vi "Configure Lister.vi"(8 "error in (no error)":errorcluster, 10 "Serial Bus Number (0: Off)":i32(ring) items=["Off", "On", "Serial Bus 1", "Serial Bus 2", "Serial Bus 3", "Serial Bus 4"], 11 "VISA resource name":refnum<visa-resource-name>) -> (0 "error out":errorcluster, 3 "VISA resource name out":refnum<visa-resource-name>)   [LabVIEW 2020, in "Agilent 90000 Series.lvlib"]
doc: "Configures the serial decode Lister."
uses:
  Agilent 90000 Series.lvlib
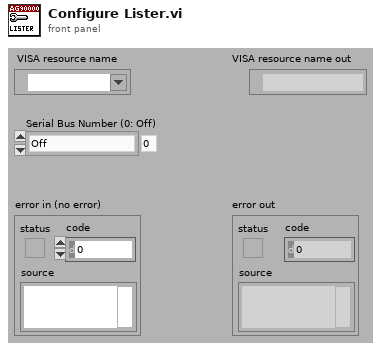
[diagram p1: front panel]
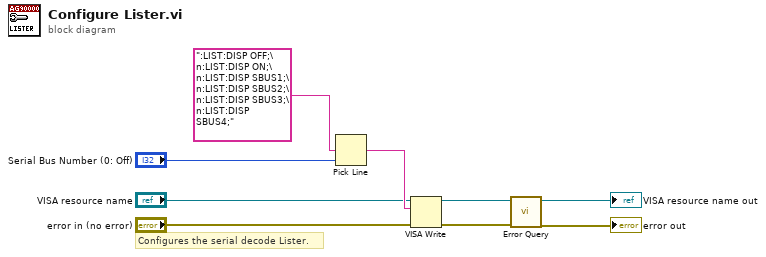
[diagram p0: block diagram]
diagram:
  # "Configures the serial decode Lister."
  n1 = Pick Line(multi-line string=":LIST:DISP OFF;\n:LIST:DISP ON;\n:LIST:DISP SBUS1;\n:LIST:DISP SBUS2;\n:LIST:DISP SBUS3;\n:LIST:DISP SBUS4;", line index="Serial Bus Number (0: Off)") -> (output string=w7:string)  [unwired: 1 out]
  n2 = VISA Write(VISA resource name="VISA resource name", write buffer=w7, error in (no error)="error in (no error)") -> (VISA resource name out=w4:refnum<visa-resource-name>, error out=w3:errorcluster)  [unwired: 1 out]
  n3 = call "Error Query.vi"("error in (no error)"=w3, "VISA resource name"=w4) -> ("error out"=→"error out":errorcluster, "VISA resource name out"=→"VISA resource name out":refnum<visa-resource-name>)  [unwired: 8 out]
